vi "ExSubSetupEMADC.vi"(0 "Camera Handle":u32, 1 "Fast ADC":bool, 2 "ReadOut Port":u32 max=1 step=1, 3 "Avalanche Gain\nOnly valid for \nport 0":dbl format="%.2f", 4 "ADC Gain":u32, 5 "error in (no error)":errorcluster) -> (6 "Camera Handle":u32, 7 "ADC Speed (Khz)":u32, 8 "error out":errorcluster)   [LabVIEW 2010]
panel:
  # "Setup EM ADC\nThis sub VI sets the\nreadout port, Avlanche\ngain, ADC (fast or slow)\nand the gain for ADC.\nIt returns the ADC speed\nselected in Khz"
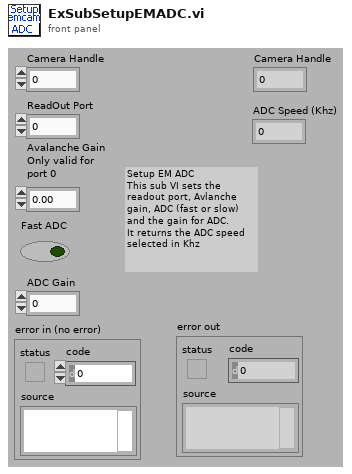
[diagram p1: front panel]
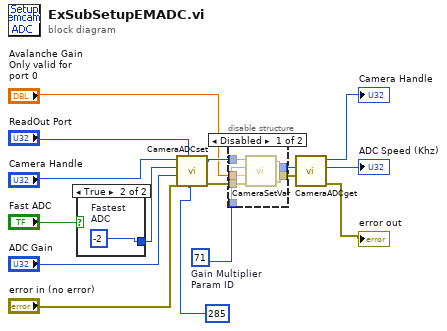
[diagram p0: block diagram]
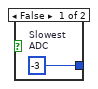
[diagram p3: hidden frame]
diagram:
  w7 = 71  # Gain Multiplier Param ID
  n1 = case shown="True" "Fast ADC" {
    tunnel: [w17 w18] -> w12
    frame False {
      w17 = -3  # Slowest ADC
    }
    frame True {
      w18 = -2  # Fastest ADC
    }
  }
  n2 = call <userlib>:"CameraADCset.vi"("ADC offset"=285, "Read Out port"="ReadOut Port", "error in (no error)"="error in (no error)", "ADC Gain"="ADC Gain", "ADC Speed"=w12, "Camera Handle"="Camera Handle") -> ("error out"=w10:errorcluster, "Camera Handle"=w9:u32)
  n3 = disable-structure shown="Disabled" {
    disable-tunnel: w10 -> [w24 _]
    disable-tunnel: w9 -> [w23 _]
    disable-tunnel: "Avalanche Gain\nOnly valid for \nport 0" -> [w22 _]
    disable-tunnel: w7 -> [w21 _]
    disable-tunnel: [w20 _] -> w6
    disable-tunnel: [w19 _] -> w5
    frame Disabled {
      n4 = call <userlib>:"CameraSetVar.vi"("error in"=w24, "Value"=w22, "Parameter ID"=w21, "Camera Handle"=w23) -> ("error out"=w20:errorcluster, "CameraHandle"=w19:u32)
    }
    frame Enabled {
    }
  }
  n5 = call <userlib>:"CameraADCget.vi"("Camera handle"=w5, "error in (no error)"=w6) -> ("Camera handle"=→"Camera Handle":u32, "ADC Speed"=→"ADC Speed (Khz)":i32, "error out"=→"error out":errorcluster)  [unwired: 5 out]
